vi "退回 最大值.vi"(11 "推力":dbl[](array[numeric])) -> (3 "最大值":dbl)   [LabVIEW 2015, in "Logging.lvlib"]
uses:
  Logging.lvlib
  <vilib>/Analysis/NI_AALPro.lvlib
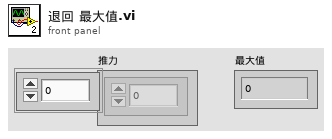
[diagram p1: front panel]
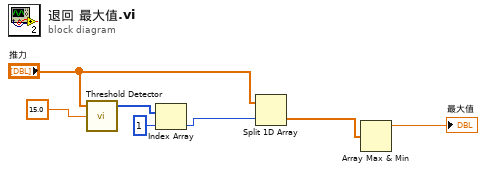
[diagram p0: block diagram]
diagram:
  n1 = call <vilib>:"Threshold Detector.vi"("threshold"=15.0, "X"="推力") -> ("Indices"=w6:i32[])  [unwired: 1 in, 2 out]
  n2 = Index Array(array=w6, index=1 ("索引")) -> (element=w4:i32)
  n3 = Split 1D Array(array="推力", index=w4) -> (second subarray=w2:dbl[])  [unwired: 1 out]
  n4 = Array Max & Min(array=w2) -> (max value=→"最大值":dbl)  [unwired: 3 out]
